vi "get sig value.vi"(8 "错误输入（无错误）":errorcluster, 9 "数据大小in":u32, 11 "信号名1in":string) -> (0 "错误输出":errorcluster, 2 "数组out":dbl[](array[numeric]))   [LabVIEW 2017]
uses:
  <userlib>/SimuLabAPIEx_V3/SimuLabAPIEx_V3.lvlib
panel:
  out "确定":bool
  in  "确定 2":bool
  in  "取消":bool
  in  "数组":dbl[](array[numeric])
  out "偏移":i32
  out "数据大小":u32
  out "信号名1":string
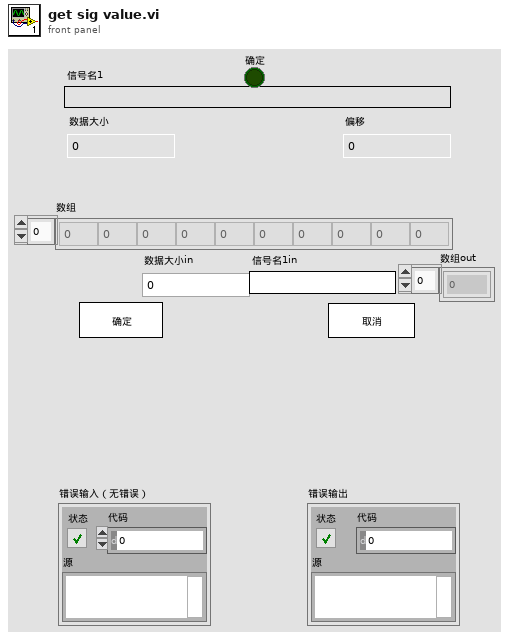
[diagram p1: front panel]
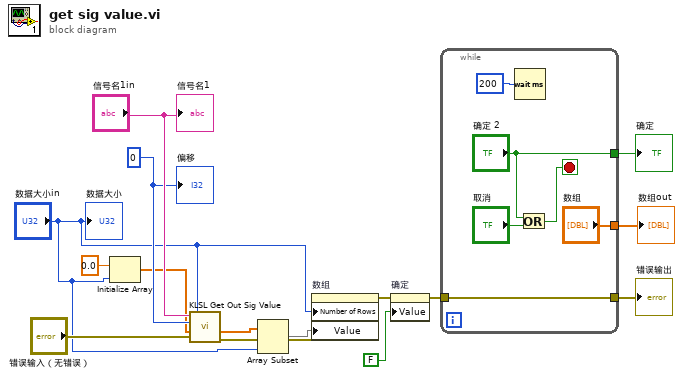
[diagram p0: block diagram]
diagram:
  w7 = 0 ("偏移")
  n1 = Initialize Array(0.0 ("元素"), "数据大小in") -> (w6:dbl[])
  n2 = call <userlib>:"KLSL Get Out Sig Value.vi"("nDataBuffLen"="数据大小in", "error in (no error)"="错误输入（无错误）", "pDataValue"=w6, "nOffSet"=w7, "szOutSigName"="信号名1in") -> ("error out"=w3:errorcluster, "pDataValue out"=w2:dbl[])  [unwired: 3 in, 2 out]
  n3 = Array Subset(array=w2, length="数据大小in") -> (w9:dbl[])  [unwired: 1 in]
  n4 = property on="数组" class="Arr (严格)"(error in=w3, "Number of Rows"="数据大小in", "Value"=w9) -> (error out=w10:errorcluster)  [unwired: 1 in, 1 out]
  n5 = property on="确定" class="Bool (严格)"(error in=w10, "Value"=FALSE ("确定")) -> (error out=w14:errorcluster)  [unwired: 1 in, 1 out]
  n6 = while {
    tunnel: ["确定 2"] -> w15
    tunnel: w14 -> [w17]
    tunnel: [w17] -> w12
    tunnel: ["数组"] -> w1
    stop <- w20 stop-if-true
    n7 = Wait (ms)(milliseconds to wait=u32 200 ("等待时间（毫秒）")) -> ()  [unwired: 1 out]
    n8 = Or(x="确定 2", y="取消") -> (x .or. y?=w20:bool)
  }
  "确定" <- w15
  "错误输出" <- w12
  "数组out" <- w1
  "信号名1" <- "信号名1in"
  "数据大小" <- "数据大小in"
  "偏移" <- w7
